vi "HttpPostRequest.vi"() -> ()   [LabVIEW 2025]
doc: "Takes student details as input from the user, makes a POST request to a specified endpoint with the input data, and stores the response in a string."
uses:
  <vilib>/httpClient/POSTBuffer.vi
  <vilib>/httpClient/LabVIEWHTTPClient.lvlib
panel:
  in  "Student":T1
  out "Response body":string
  # "Take student details as input from user and make post request and store the response in a string"
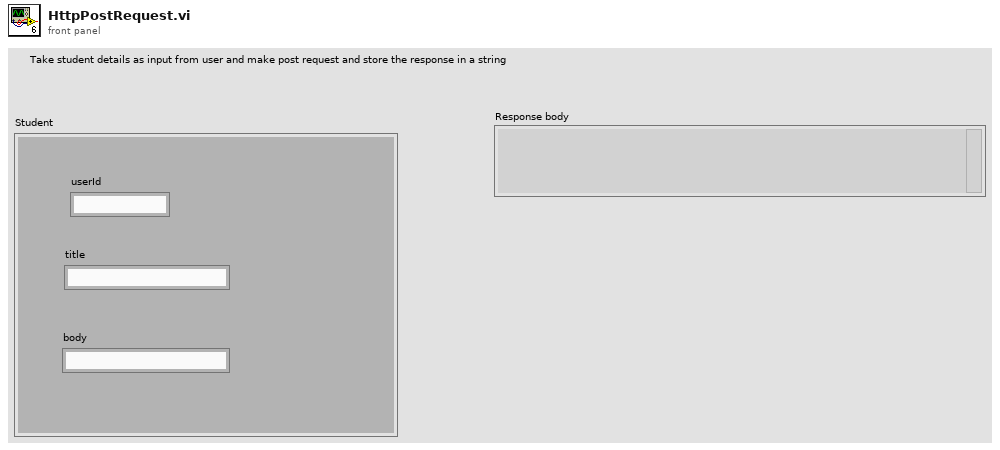
[diagram p1: front panel]
types:
  T1 = cluster{"userId":string, "title":string, "body":string}
  T2 = typedef "LabVIEWHTTPClient.lvlib/ClientHandle.ctl" = refnum<k1>
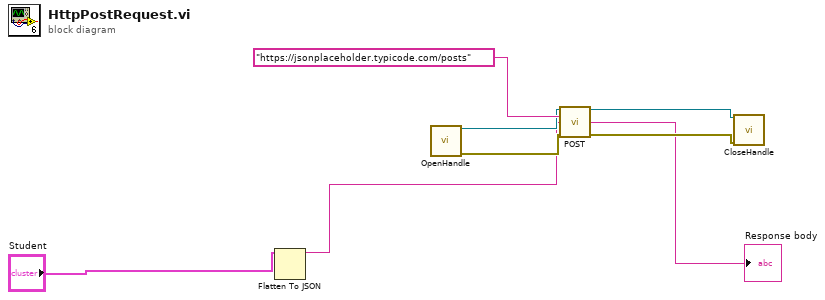
[diagram p0: block diagram]
diagram:
  n1 = Flatten To JSON(anything="Student") -> (JSON string=w3:string)  [unwired: 2 in, 1 out]
  n2 = call <vilib>:"OpenHandle.vi"() -> ("client handle out"=w6:T2, "error out"=w7:errorcluster)  [unwired: 14 in]
  n3 = call-poly <vilib>:"POST.vi"("client handle"=w6, "url"="https://jsonplaceholder.typicode.com/posts", "buffer"=w3, "error in (no error)"=w7) -> ("client handle out"=w5:T2, "body"=→"Response body":string, "error out"=w4:errorcluster)  [unwired: 8 in, 1 out]
  n4 = call <vilib>:"CloseHandle.vi"("client handle"=w5, "error in (no error)"=w4) -> ()  [unwired: 13 in, 1 out]
